vi "Initialize Script UI.vi"(8 "error in":errorcluster, 10 "Script UI Ctrl Ref":T2, 11 "Script Meas Config Ctrl Ref":T1) -> (0 "error out":errorcluster)   [LabVIEW 2025, in "Fgen Script Mode UI.lvlib"]
uses:
  Fgen Script Mode UI.lvlib
  Typedef/Script Meas Config Ctrl Ref.ctl
  Typedef/Script UI Ctrl Ref.ctl
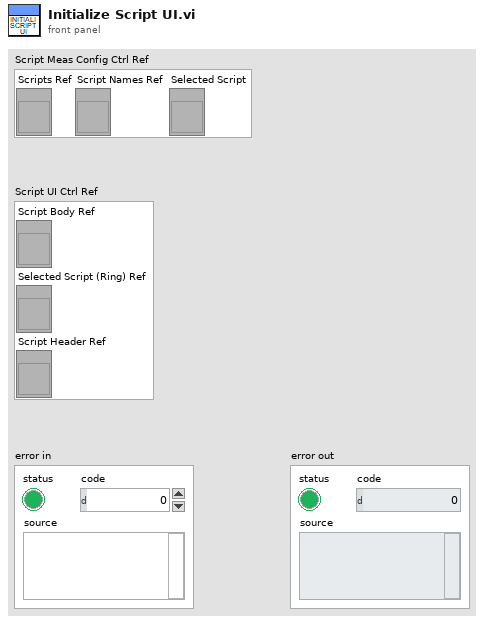
[diagram p1: front panel]
types:
  T1 = typedef "Fgen Script Mode UI.lvlib/Script Meas Config Ctrl Ref.ctl" = cluster{"Scripts Ref":refnum<vi>, "Script Names Ref":refnum<vi>, "Selected Script":refnum<vi>}
  T2 = typedef "Fgen Script Mode UI.lvlib/Script UI Ctrl Ref.ctl" = cluster{"Script Body Ref":refnum<vi>, "Selected Script (Ring) Ref":refnum<vi>, "Script Header Ref":refnum<vi>}
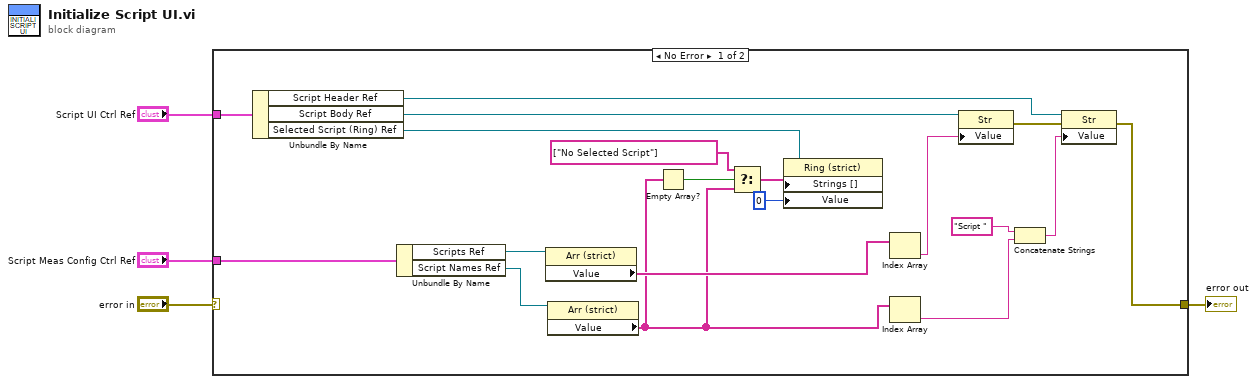
[diagram p0: block diagram]
diagram:
  n1 = case shown="No Error" "error in" {
    selector: "error in" -> [_ w24]
    tunnel: [w14 w24] -> w3
    tunnel: "Script Meas Config Ctrl Ref" -> [w21 _]
    tunnel: "Script UI Ctrl Ref" -> [w23 _]
    frame No Error {
      n2 = Unbundle By Name(w23) -> ("Script Header Ref"=w13:refnum<vi>, "Script Body Ref"=w19:refnum<vi>, "Selected Script (Ring) Ref"=w22:refnum<vi>)
      n3 = Unbundle By Name(w21) -> ("Scripts Ref"=w20:refnum<vi>, "Script Names Ref"=w15:refnum<vi>)
      n4 = property class="Arr (strict)"(reference=w20) -> ("Value"=w18:string[])  [unwired: 1 in, 2 out]
      n5 = property class="Arr (strict)"(reference=w15) -> ("Value"=w6:string[])  [unwired: 1 in, 2 out]
      n6 = Empty Array?(array=w6) -> (empty?=w7:bool)
      n7 = Select(t=string[] ["No Selected Script"], s=w7, f=w6) -> (s? t:f=w8:string[])
      n8 = property class="Ring (strict)"(reference=w22, "Strings []"=w8, "Value"=u16 0) -> ()  [unwired: 1 in, 2 out]
      n9 = Index Array(array=w18) -> (element=w17:string)  [unwired: 1 in]
      n10 = Index Array(array=w6) -> (element=w11:string)  [unwired: 1 in]
      n11 = property class="Str"(reference=w19, "Value"=w17) -> (error out=w16:errorcluster)  [unwired: 1 in, 1 out]
      n12 = Concatenate Strings("Script " ("string"), w11) -> (w10:string)
      n13 = property class="Str"(reference=w13, error in=w16, "Value"=w10) -> (error out=w14:errorcluster)  [unwired: 1 out]
    }
    frame Error {
    }
  }
  "error out" <- w3
